vi "Reading_ELYs_OPC_UA (SubVI).vi"(5 "milliseconds to wait":u32=500, 6 "Array 4":refnum<vi>[][](array[refnum]), 8 "error in (no error)":errorcluster, 9 "ELYs in":map{string, dbl}[](array[numeric]), 10 "ELYs to read":string[](array[string])=["1.1", "1.2", "1.3", "2.1", "2.2", "2.3"], 11 "Refnum in":T1) -> (0 "error out":errorcluster, 2 "ELYs out":map{string, dbl}[](array[numeric]), 3 "Refnum out":T1)   [LabVIEW 2024]
uses:
  <vilib>/OPCUA/controls/OPC UA Client Refnum.ctl
  S7-1200_OPCUA.lvlib
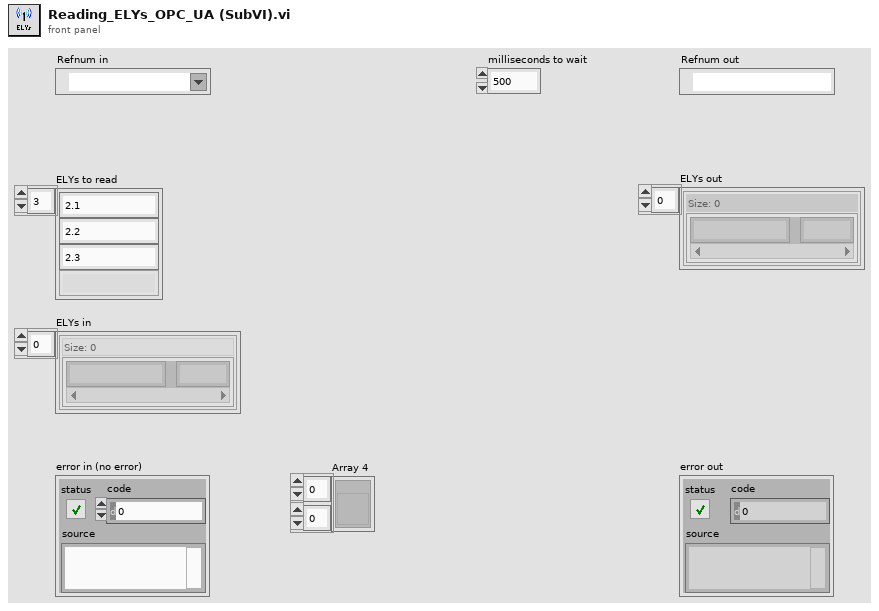
[diagram p1: front panel]
types:
  T1 = typedef "OPC UA Client Refnum.ctl" = refnum<k21>
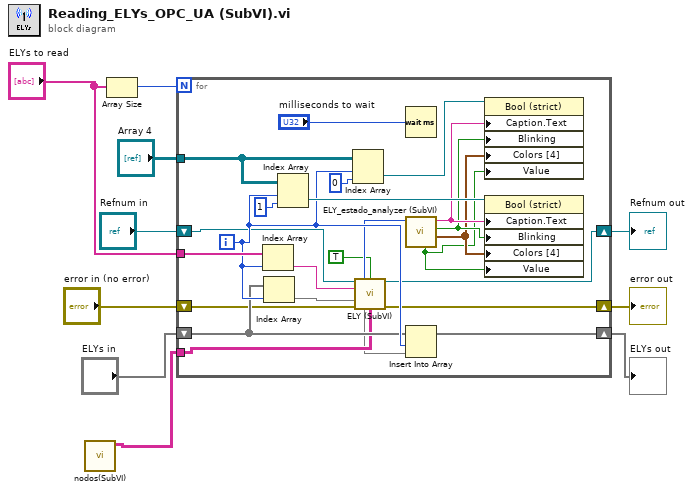
[diagram p0: block diagram]
diagram:
  n1 = call "nodos(SubVI).vi"() -> ("Array"=w1:string[][])  [unwired: 11 in]
  n2 = Array Size(array="ELYs to read") -> (size(s)=w2:i32)
  n3 = for {
    N: w2 -> [_]
    shift-right: [w16] -> w6
    shift-left: "Refnum in" -> [w19]
    shift-right: [w15] -> w10
    shift-left: "error in (no error)" -> [w18]
    tunnel: "ELYs to read" -> [w34]
    tunnel: "Array 4" -> [w33]
    shift-right: [w22] -> w9
    shift-left: "ELYs in" -> [w23]
    tunnel: w1 -> [w21]
    i -> [w24]
    n4 = Index Array(array=w34, index=w24) -> (element=w20:string)
    n5 = Index Array(array=w23, index=w24) -> (element=w17:map{string, dbl})
    n6 = Index Array(array=w33, index (row)=w24, index (col)=1 ("disabled index (col)")) -> (element=w29:refnum<vi>)
    n7 = Index Array(array=w33, index (row)=w24, index (col)=0 ("disabled index (col)")) -> (element=w30:refnum<vi>)
    n8 = call "ELY (SubVI).vi"("Refnum in"=w19, "Leer mas¿?"=TRUE, "Electrolizador"=w20, "Medidas in"=w17, "error in (no error)"=w18, "Nodos"=w21) -> ("Estado"=w13:u16, "Refnum out"=w16:T1, "Medidas"=w14:map{string, dbl}, "error out"=w15:errorcluster)  [unwired: 3 in, 3 out]
    n9 = Wait (ms)(milliseconds to wait="milliseconds to wait") -> ()  [unwired: 1 out]
    n10 = call "ELY_estado_analyzer (SubVI).vi"("Numeric"=w13) -> ("Colors [4]"=w26:cluster{u32, u32}[], "Boolean 2"=w27:bool, "Caption.Text"=w28:string, "Boolean"=w25:bool)  [unwired: 7 in]
    n11 = Insert Into Array(array=w23, index=w24, new element=w14) -> (w22:map{string, dbl}[])
    n12 = property class="Bool (strict)"(reference=w30, "Caption.Text"=w28, "Blinking"=w27, "Colors [4]"=w26, "Value"=w25) -> ()  [unwired: 1 in, 2 out]
    n13 = property class="Bool (strict)"(reference=w29, "Caption.Text"=w28, "Blinking"=w27, "Colors [4]"=w26, "Value"=w25) -> ()  [unwired: 1 in, 2 out]
  }
  "error out" <- w10
  "ELYs out" <- w9
  "Refnum out" <- w6
